vi "save min value.vi"(4 "State":i16, 5 "Time":dbl format="%.2f", 6 "Sensor Values":dbl[](array[numeric]), 7 "Set Points":dbl[](array[numeric])) -> (0 "required data":T1={"Set Point names"=["x value to save", "state to save"], "required number of setpoints"=2, "required number of sensors"=1, "Sensor names"=["sensor to save"]}, 3 "output value":dbl)   [LabVIEW 2012]
panel:
  in  "Path":path=path "C:/data/state_min_values.xls"
  # "Enter the correct information for this control code in the required data structure below. Then make the current value default by right clicking on the border of the data structure. Select \"data operations\" and then select \"make current value default\". These values will be displayed by process controller."
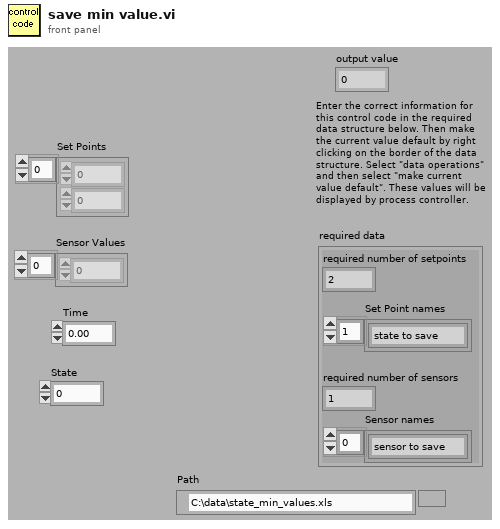
[diagram p1: front panel]
types:
  T1 = cluster{"Set Point names":string[], "required number of setpoints":u8, "required number of sensors":u8, "Sensor names":string[]}
  T2 = enum16{"open", "open or create", "create or replace", "create", "open (read only)"}
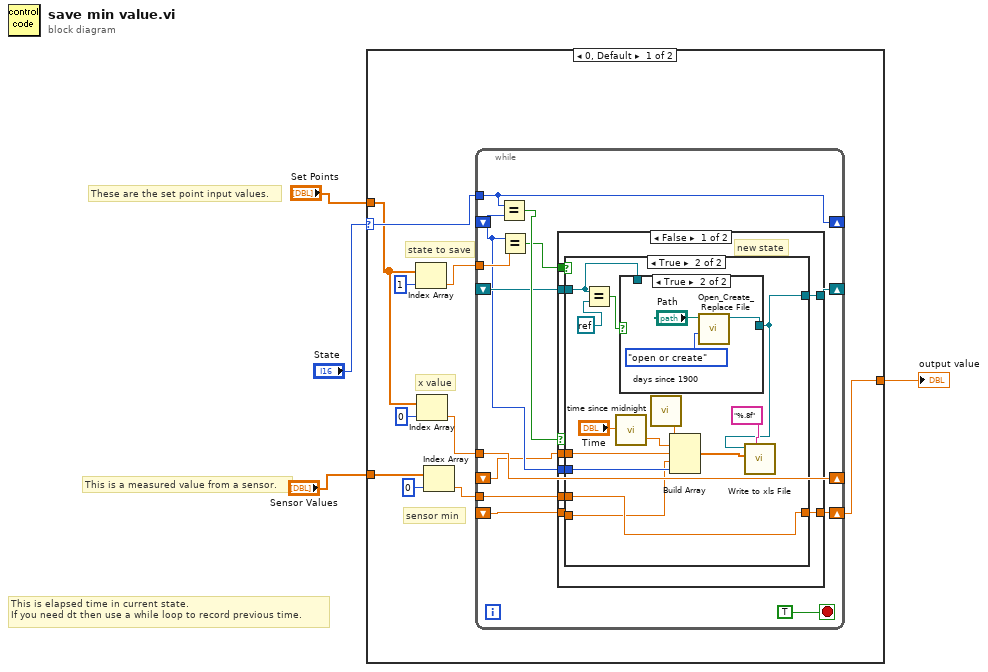
[diagram p0: block diagram]
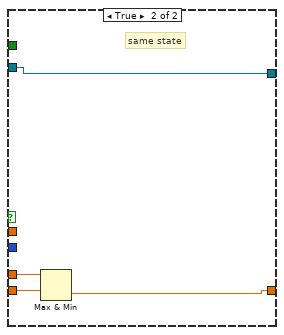
[diagram p4: hidden frame]
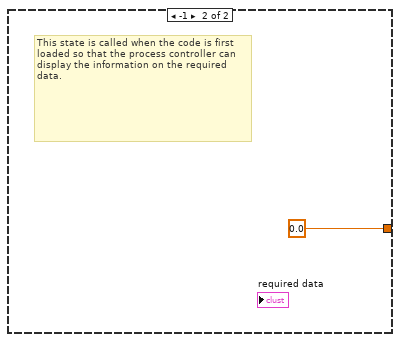
[diagram p5: hidden frame]
diagram:
  # "These are the set point input values."
  # "This is a measured value from a sensor."
  # "This is elapsed time in current state.\nIf you need dt then use a while loop to record previous time."
  n1 = case shown="0, Default" "State" {
    selector: "State" -> [w11 _]
    tunnel: [w8 0.0 ("fraction on")] -> w3
    tunnel: "Set Points" -> [w6 _]
    tunnel: "Sensor Values" -> [w12 _]
    frame 0, Default {
      # "x value"
      # "state to save"
      # "sensor min"
      n2 = Index Array(array=w6, index=1) -> (element=w10:dbl)
      n3 = Index Array(array=w6, index=0) -> (element=w5:dbl)
      n4 = Index Array(array=w12, index=0) -> (element=w9:dbl)
      n5 = while {
        shift-right: [w23] -> w8
        shift-left: _ -> [w25]
        shift-right: [w26] -> _
        shift-left: _ -> [w17]
        tunnel: w11 -> [w26]
        tunnel: w10 -> [w18]
        tunnel: w9 -> [w24]
        shift-right: [w20] -> _
        shift-left: _ -> [w19]
        tunnel: w5 -> [w16]
        shift-right: [w16] -> _
        shift-left: _ -> [w15]
        stop <- TRUE stop-if-true
        n6 = Equal?(x=w26, y=w17) -> (x = y?=w22:bool)
        n7 = Equal?(x=w17, y=w18) -> (x = y?=w21:bool)
        n8 = case shown="False" w22 {
          tunnel: w25 -> [w35 w57]
          tunnel: w24 -> [w34 w58]
          tunnel: [w33 w56] -> w23
          tunnel: w21 -> [w32 _]
          tunnel: w17 -> [w31 _]
          tunnel: [w30 w55] -> w20
          tunnel: w19 -> [w29 w55]
          tunnel: w15 -> [w28 _]
          frame False {
            # "new state"
            n9 = case shown="True" w32 {
              tunnel: w35 -> [_ w41]
              tunnel: w34 -> [w37 w50]
              tunnel: [w37 w50] -> w33
              tunnel: w31 -> [_ w42]
              tunnel: [w36 w46] -> w30
              tunnel: w29 -> [w36 w43]
              tunnel: w28 -> [_ w40]
              frame False {
              }
              frame True {
                n10 = Equal?(x=w43, y=refnum<k0> refnum) -> (x = y?=w45:bool)
                n11 = call "time since midnight.vi"("seconds since 1Jan1904"="Time") -> ("Days"=w39:dbl)  [unwired: 1 out]
                n12 = case shown="True" w45 {
                  tunnel: [w51 w52] -> w46
                  tunnel: w43 -> [w51 _]
                  frame False {
                  }
                  frame True {
                    n13 = call <vilib>:"Open_Create_Replace File.vi"("function (open:0)"=T2."open or create", "file path"="Path") -> ("refnum"=w52:refnum<file>)  [unwired: 6 in, 3 out]
                  }
                }
                n14 = call "days since 1900.vi"() -> ("Days"=w38:dbl)  [unwired: 1 in]
                n15 = Build Array(w38, w39, w40, w41, w42) -> (w48:dbl[])
                n16 = call "Write to xls File.vi"("format (%.3f)"="%.8f", "1D data"=w48, "refnum"=w46) -> ()  [unwired: 7 in, 2 out]
              }
            }
          }
          frame True {
            # "same state"
            n17 = Max & Min(x=w58, y=w57) -> (min(x,y)=w56:dbl)  [unwired: 1 out]
          }
        }
      }
    }
    frame -1 {
      # "This state is called when the code is first loaded so that the process controller can display the information on the required data."
    }
  }
  "output value" <- w3
